vi "PushToErrorHandler.vi"(0 "ErrorIn":errorcluster, 1 "ErrorLocation":string) -> (5 "ErrorOut":errorcluster)   [LabVIEW 2018]
doc: "When <B>ErrorIn</B> contains an error condition, place the error into <B>ClusterIn</B>'s queue member \"Q\".\n\nThe Main (Consumer) Loop dequeues this error and takes appropriate action depending on the error.\n\nCopyright © 2019 Epimedia, Inc. All Rights Reserved.\n\nThe Epimedia Application Library is Copyright © 2009-2017 Epimedia, Inc. \nAll Rights Reserved. Used under license."
uses:
  Queue/MainQueueElements.ctl
panel:
  # "Copyright © 2019 Epimedia, Inc. All Rights Reserved.\n\nThe Epimedia Application Library is Copyright © 2009-2017 Epimedia, Inc. \nAll Rights Reserved. Used under license."
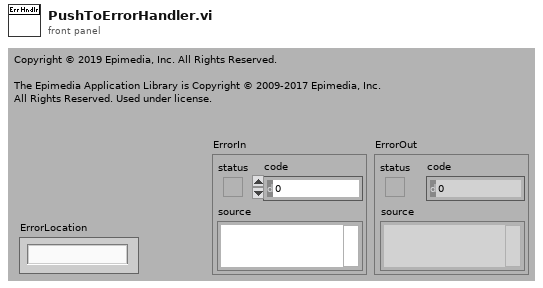
[diagram p1: front panel]
types:
  T1 = typedef "MainQueueElements.ctl" = enum16{"Spvsr_InitQ", "Spvsr_RfrshPnl", "Spvsr_InitSW", "Spvsr_InitCtrls", "Spvsr_Cursors", "Spvsr_StrtHWLp", "Spvsr_Stop", "Spvsr_NewData", "Spvsr_ScaleGraphs", "Spvsr_Error", "Spvsr_About", "Spvsr_Config", "Spvsr_FPConfig", "Spvsr_AlarmCfg", "Spvsr_DigitzOffs", "FP_AO_ctrl", "Spvsr_RestartWarn", "Spvsr_AutoCenter", "Spvsr_TrackRate", "Spvsr_ChkTime", "Spvsr_Admin", "Spvsr_Exit"}
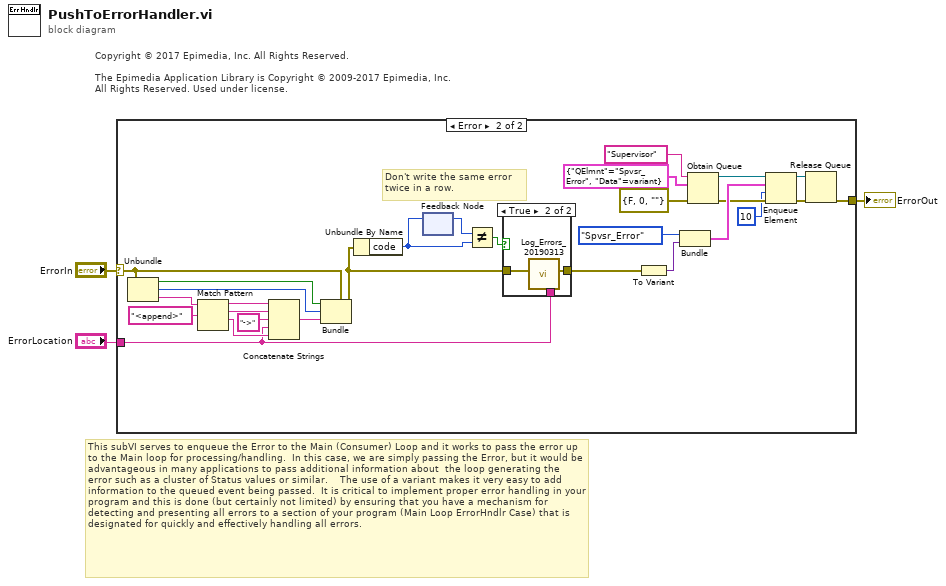
[diagram p0: block diagram]
diagram:
  # "This subVI serves to enqueue the Error to the Main (Consumer) Loop and it works to pass the error up to the Main loop for processing/handling.  In this case, we are simply passing the Error, but it would be advantageous in many applications to pass additional information about  the loop generating the error such as a cluster of Status values or similar.    The use of a variant makes it very easy to add information to the queued event being passed.  It is critical to implement proper error handling in your program and this is done (but certainly not limited) by ensuring that you have a mechanism for detecting and presenting all errors to a section of your program (Main Loop ErrorHndlr Case) that is designated for quickly and effectively handling all errors."
  # "Copyright © 2017 Epimedia, Inc. All Rights Reserved.\n\nThe Epimedia Application Library is Copyright © 2009-2017 Epimedia, Inc. \nAll Rights Reserved. Used under license."
  n1 = case shown="Error" "ErrorIn" {
    selector: "ErrorIn" -> [w4 w19]
    tunnel: [w4 w31] -> w3
    tunnel: "ErrorLocation" -> [_ w10]
    frame No Error {
    }
    frame Error {
      # "Don't write the same error \ntwice in a row."
      n2 = Unbundle(w19) -> ("status"=w27:bool, "code"=w26:i32, "source"=w18:string)
      n3 = Match Pattern(string=w18, regular expression="<append>") -> (before substring=w24:string, match substring=w23:string, after substring=w22:string)  [unwired: 1 in, 1 out]
      n4 = Concatenate Strings(w24, w23, "->" ("string"), w10, w22) -> (w20:string)
      n5 = Bundle(cluster=w19, "status"=w27, "code"=w26, "source"=w20) -> (w8:errorcluster)
      n6 = Unbundle By Name(w8) -> ("code"=w7:i32)
      n7 = feedback-in #1(w7) -> ()
      n8 = feedback #1() -> (w6:i32)  [unwired: 1 in]
      n9 = Not Equal?(x=w6, y=w7) -> (x != y?=w5:bool)
      n10 = case shown="True" w5 {
        tunnel: [w32 w35] -> w11
        tunnel: w10 -> [_ w34]
        tunnel: w8 -> [w32 w33]
        frame False {
        }
        frame True {
          n11 = call "Log_Errors_20190313.vi"("LoopName"=w34, "error in"=w33) -> ("error out"=w35:errorcluster)  [unwired: 9 in]
        }
      }
      n12 = To Variant(anything=w11) -> (Variant=w29:variant)
      n13 = Bundle("QElmnt"=MainQueueElements."Spvsr_Error", "Variant"=w29) -> (w28:cluster{"QElmnt":T1, "Variant":variant})  [unwired: 1 out]
      n14 = Obtain Queue(name (unnamed)="Supervisor", element data type=cluster{"QElmnt":T1, "Data":variant} {"QElmnt"=enum."Spvsr_Error", "Data"=variant} ("Cluster"), error in (no error)=errorcluster {"status"=FALSE, "code"=0, "source"=""} ("error IO")) -> (queue out=w16:refnum<queue>, error out=w14:errorcluster)  [unwired: 2 in, 1 out]
      n15 = Enqueue Element(queue=w16, element=w28, timeout in ms (-1)=10, error in (no error)=w14) -> (queue out=w13:refnum<queue>, error out=w31:errorcluster)  [unwired: 1 out]
      n16 = Release Queue(queue=w13) -> ()  [unwired: 2 in, 3 out]
    }
  }
  "ErrorOut" <- w3
